vi "set_output_on.vi"(8 "error in":errorcluster, 11 "VISA resource name":refnum<visa-resource-name>="COM1") -> (0 "error out":errorcluster, 3 "VISA resource name out":refnum<visa-resource-name>)   [LabVIEW 2020]
panel:
  out "command":string
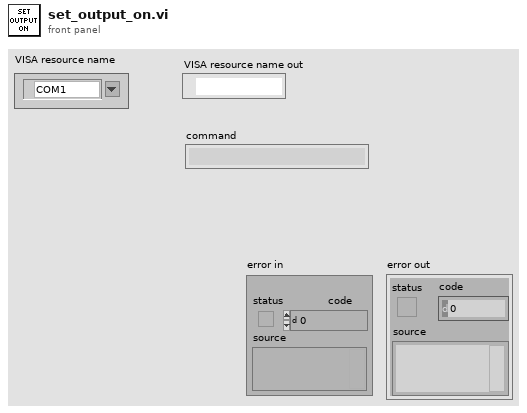
[diagram p1: front panel]
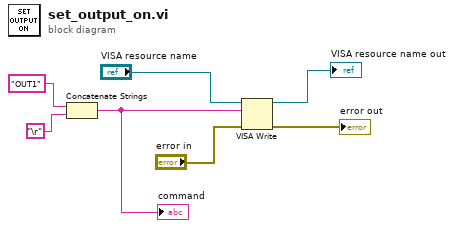
[diagram p0: block diagram]
diagram:
  n1 = Concatenate Strings("OUT1" ("string"), "\r") -> (w2:string)
  "command" <- w2
  n2 = VISA Write(VISA resource name="VISA resource name", write buffer=w2, error in (no error)="error in") -> (VISA resource name out=→"VISA resource name out":refnum<visa-resource-name>, error out=→"error out":errorcluster)  [unwired: 1 out]
